vi "SAE J-1939 Signalliste Text.vi"(8 "Fehler (Eingang, kein Fehler)":errorcluster, 11 "Referenz (Eingang)":refnum<k21>) -> (0 "Fehler (Ausgang)":errorcluster, 2 "Signal IDs Array":T1(array[cluster]), 3 "SAE J-1939 Signal-Cluster":T2[](array[typedef]), 4 "Signal IDs Array Größe(n)":i32, 5 "SAE J-1939 Signal-Cluster Größe(n)":i32)   [LabVIEW 2020, in "OBD Daten.lvlib"]
uses:
  OBD Daten.lvlib
  SAE J-1938 Signal.ctl
  <resource>/objmgr/xnet.rc
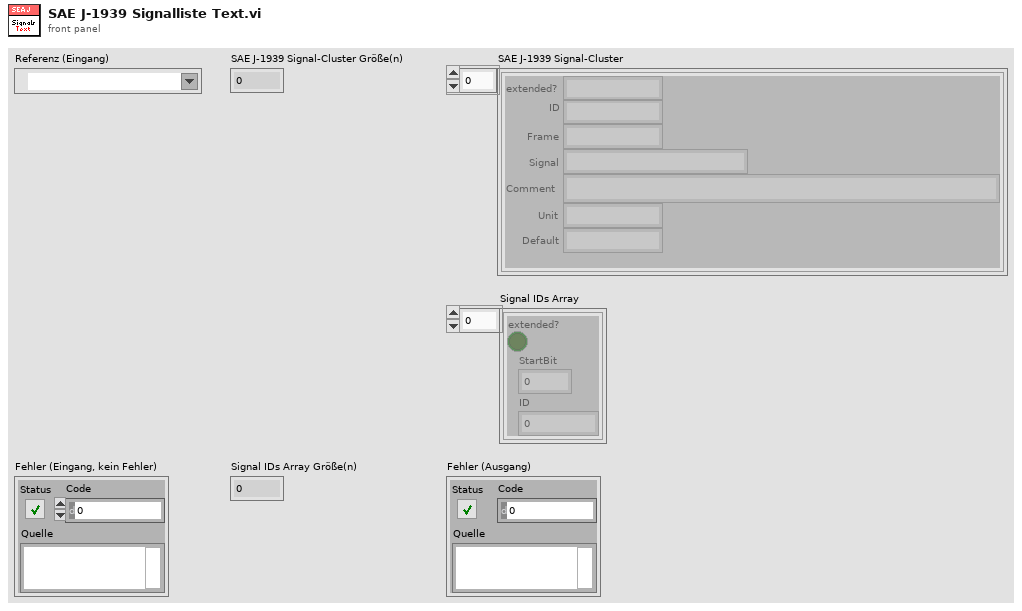
[diagram p1: front panel]
types:
  T1 = cluster{"extended?":bool, "StartBit":u32, "ID":u32}[]
  T2 = typedef "OBD Daten.lvlib/SAE J-1938 Signal.ctl" = cluster{"extended?":string, "ID":string, "Frame":string, "Signal":string, "Comment":string, "Unit":string, "Default":string}
  T3 = cluster{"CAN.ExtID?":bool, "StartBit":u32, "ID":u32}[]
  T4 = cluster{"CAN.ExtID?":bool, "StartBit":u32, "ID":u32}
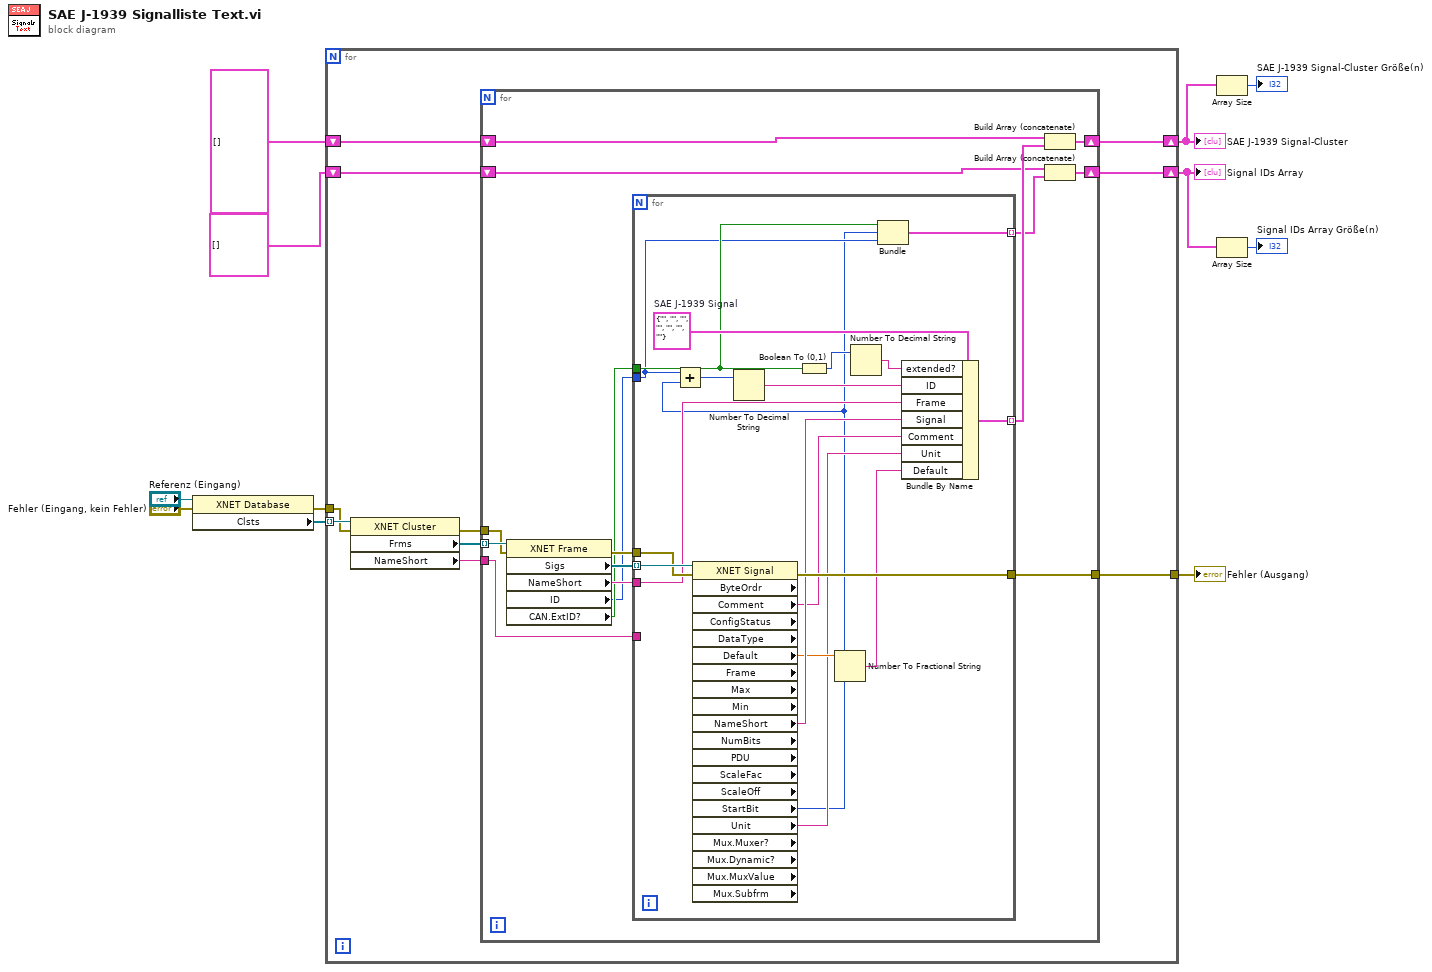
[diagram p0: block diagram]
diagram:
  n1 = property class="XNET Database"(reference="Referenz (Eingang)", error in="Fehler (Eingang, kein Fehler)") -> (error out=w9:errorcluster, "Clsts"=w11:refnum<k21>[])  [unwired: 1 out]
  n2 = for {
    tunnel: w11 -> [w21] mode=indexing
    tunnel: w9 -> [w19]
    tunnel: [w17] -> w7
    shift-right: [w15] -> w3
    shift-left: T2[] [] -> [w14]
    shift-right: [w13] -> w4
    shift-left: T3 [] -> [w12]
    n3 = property class="XNET Cluster"(reference=w21, error in=w19) -> (error out=w18:errorcluster, "Frms"=w20:refnum<k21>[], "NameShort"=w16:string)  [unwired: 1 out]
    n4 = for {
      tunnel: w20 -> [w36] mode=indexing
      tunnel: w18 -> [w34]
      tunnel: [w32] -> w17
      tunnel: w16 -> [w30]
      shift-right: [w25] -> w15
      shift-left: w14 -> [w26]
      shift-right: [w23] -> w13
      shift-left: w12 -> [w22]
      n5 = property class="XNET Frame"(reference=w36, error in=w34) -> (error out=w33:errorcluster, "Sigs"=w35:refnum<k21>[], "NameShort"=w31:string, "ID"=w28:u32, "CAN.ExtID?"=w29:bool)  [unwired: 1 out]
      n6 = for {
        tunnel: w35 -> [w55] mode=indexing
        tunnel: w33 -> [w54]
        tunnel: [w53] -> w32
        tunnel: w31 -> [w50]
        tunnel: w30 -> [_]
        tunnel: w29 -> [w41]
        tunnel: w28 -> [w40]
        tunnel: [w44] -> w27 mode=indexing
        tunnel: [w39] -> w24 mode=indexing
        w52 = T2 {"extended?"="", "ID"="", "Frame"="", "Signal"="", "Comment"="", "Unit"="", "Default"=""}  # SAE J-1939 Signal
        n7 = property class="XNET Signal" props=["ByteOrdr", "Comment", "ConfigStatus", "DataType", "Default", "Frame", "Max", "Min", "NameShort", "NumBits", "PDU", "ScaleFac", "ScaleOff", "StartBit", "Unit", "Mux.Muxer?", "Mux.Dynamic?", "Mux.MuxValue", "Mux.Subfrm"](reference=w55, error in=w54) -> (error out=w53:errorcluster, "Comment"=w48:string, "Default"=w47:dbl, "NameShort"=w49:string, "StartBit"=w37:u32, "Unit"=w46:string)  [unwired: 15 out]
        n8 = Add(x=w40, y=w37) -> (x+y=w38:u32)
        n9 = Number To Decimal String(number=w38) -> (decimal integer string=w51:string)  [unwired: 1 in]
        n10 = Boolean To (0,1)(Boolean=w41) -> (0, 1=w43:i16)
        n11 = Number To Fractional String(number=w47) -> (F-format string=w45:string)  [unwired: 3 in]
        n12 = Number To Decimal String(number=w43) -> (decimal integer string=w42:string)  [unwired: 1 in]
        n13 = Bundle("CAN.ExtID?"=w41, "StartBit"=w37, "ID"=w40) -> (w39:T4)  [unwired: 1 in]
        n14 = Bundle By Name(cluster=w52, "extended?"=w42, "ID"=w51, "Frame"=w50, "Signal"=w49, "Comment"=w48, "Unit"=w46, "Default"=w45) -> (w44:T2)
      }
      n15 = Build Array (concatenate)(w26, w27) -> (w25:T2[])
      n16 = Build Array (concatenate)(w22, w24) -> (w23:T3)
    }
  }
  "Fehler (Ausgang)" <- w7
  "SAE J-1939 Signal-Cluster" <- w3
  "Signal IDs Array" <- w4
  n17 = Array Size(array=w3) -> (size(s)=→"SAE J-1939 Signal-Cluster Größe(n)":i32)
  n18 = Array Size(array=w4) -> (size(s)=→"Signal IDs Array Größe(n)":i32)
